vi "uninitialize.vi"(8 "error in":errorcluster, 9 "Timeout (ms)":i32=-1, 11 "profibus reference":T1) -> (0 "error out":errorcluster, 3 "profibus reference out":T1)   [LabVIEW 2013, in "dynamic profibus.lvlib"]
uses:
  dynamic profibus.lvlib
  <vilib>/rvi/interface/nirviMethod/nirviMethod.xnode
  profibus master action.ctl
  fpga reference.ctl
  <vilib>/FPGAPlugInAG/Dynamic/niLvFpga_WriteFifo_Dynamic.vi
  <vilib>/rvi/errors/niLvFpgaMergeErrorWithErrorCode.vi
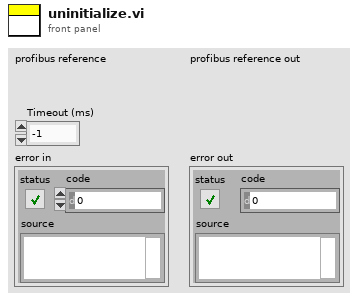
[diagram p1: front panel]
types:
  T1 = typedef "dynamic profibus.lvlib/fpga reference.ctl" = refnum<k20>
  T2 = typedef "dynamic profibus.lvlib/profibus master action.ctl" = enum8{"initialize", "uninitialize", "stop", "get input", "get input size", "set output", "get output size", "get diagnostic", "transfer data", "transfer diagnostics", "read many inputs"}
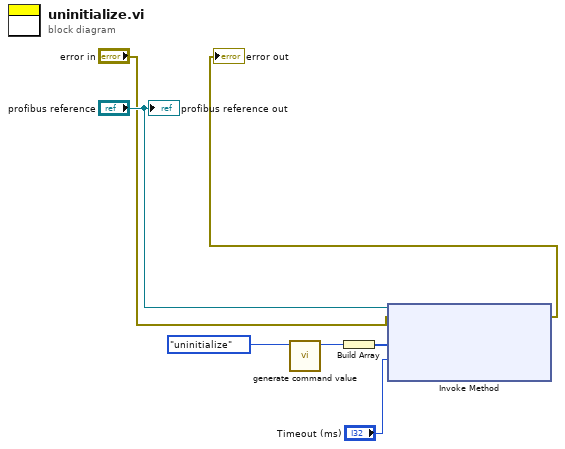
[diagram p0: block diagram]
diagram:
  n1 = call "generate command value.vi"("action"=profibus_master_action."uninitialize") -> ("Element"=w6:u32)  [unwired: 10 in]
  n2 = Build Array(w6) -> (w5:u32[])
  n3 = xnode "Invoke Method"("FPGA VI Reference In"="profibus reference", "error in"="error in", "Data"=w5, "Timeout (ms)"="Timeout (ms)") -> ("error out"=→"error out":errorcluster)  [unwired: 2 out]
  "profibus reference out" <- "profibus reference"
